vi "TCP-IP Q_Bridge.VerifyHandShake.vi"(11 "Msg In":string) -> (2 "OK":bool, 3 "Msg Out":string)   [LabVIEW 2024, in "EQMF.lvlib" / "TCP-IP.lvlib"]
uses:
  TCP-IP.lvlib
panel:
  out "Pos In":u32
  out "Pos Out":i32
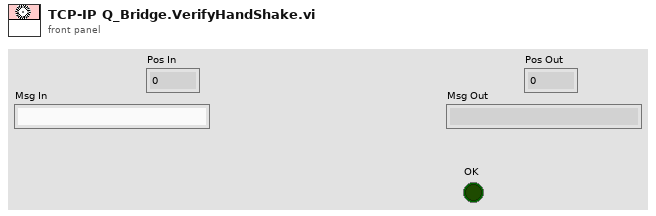
[diagram p1: front panel]
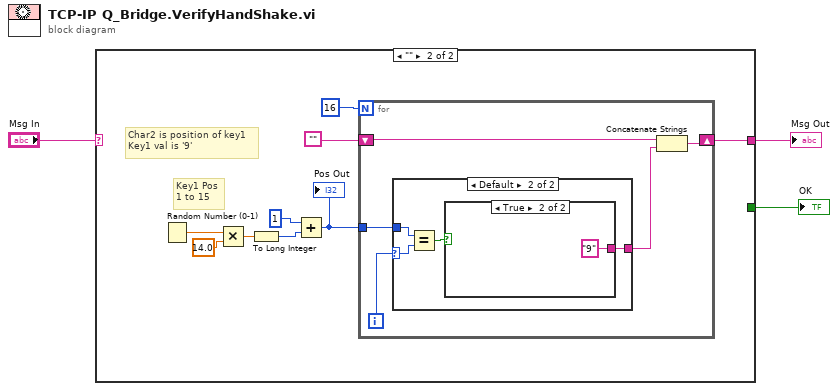
[diagram p0: block diagram]
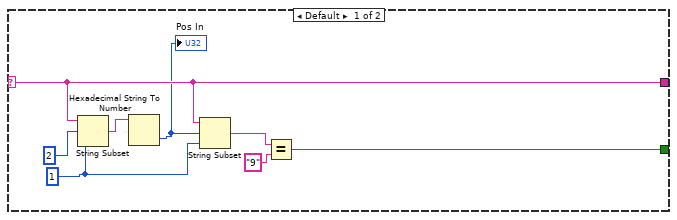
[diagram p2: hidden frame]
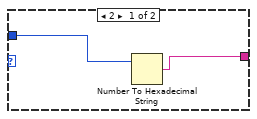
[diagram p3: hidden frame]
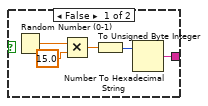
[diagram p4: hidden frame]
diagram:
  n1 = case shown="\"\"" "Msg In" {
    selector: "Msg In" -> [w9 _]
    tunnel: [w9 w19] -> w3
    tunnel: [w4 _] -> w1
    frame Default {
      w8 = 1 ("length (rest)")
      n2 = String Subset(string=w9, offset (0)=2, length (rest)=w8) -> (substring=w10:string)
      n3 = Hexadecimal String To Number(string=w10) -> (number=w7:u32)  [unwired: 2 in, 1 out]
      "Pos In" <- w7
      n4 = String Subset(string=w9, offset (0)=w7, length (rest)=w8) -> (substring=w6:string)
      n5 = Equal?(x=w6, y="9") -> (x = y?=w4:bool)
    }
    frame "" {
      # "Char2 is position of key1\nKey1 val is '9'"
      # "Key1 Pos\n1 to 15"
      n6 = Random Number (0-1)() -> (number: 0 to 1=w17:dbl)
      n7 = Multiply(x=w17, y=14.0) -> (x*y=w18:dbl)
      n8 = To Long Integer(number=w18) -> (32bit integer=w15:i32)
      n9 = Add(x=1, y=w15) -> (x+y=w12:i32)
      "Pos Out" <- w12
      n10 = for {
        N: 16 -> [_]
        shift-right: [w25] -> w19
        shift-left: "" -> [w24]
        tunnel: w12 -> [w21]
        i -> [w22]
        n11 = case shown="Default" w22 {
          selector: w22 -> [_ w28]
          tunnel: [w26 w31] -> w23
          tunnel: w21 -> [w27 w29]
          frame 2 {
            n12 = Number To Hexadecimal String(2:w27) -> (0:w26:string)  [unwired: 1 in]
          }
          frame Default {
            n13 = Equal?(x=w29, y=w28) -> (x = y?=w30:bool)
            n14 = case shown="True" w30 {
              tunnel: [w32 "9"] -> w31
              frame False {
                n15 = Random Number (0-1)() -> (number: 0 to 1=w35:dbl)
                n16 = Multiply(x=w35, y=15.0) -> (x*y=w34:dbl)
                n17 = To Unsigned Byte Integer(number=w34) -> (unsigned 8bit integer=w33:u8)
                n18 = Number To Hexadecimal String(2:w33) -> (0:w32:string)  [unwired: 1 in]
              }
              frame True {
              }
            }
          }
        }
        n19 = Concatenate Strings(w24, w23) -> (w25:string)
      }
    }
  }
  "Msg Out" <- w3
  "OK" <- w1
